vi "Init Chnl from CnfgFile.vi"(8 "error in (no error)":errorcluster, 10 "ChnlSettings":T1={"Channel Name"="", "ChnParameter"={" Delay (µs)"=0.0, "On?"=FALSE, "PositiveVoltage?"=FALSE, "50OhmTerminated? "=FALSE, "25OhmOutput?"=FALSE}, "DelayFormula"="", "OutputModulo"=1, "Go and Done Signal"={"Go Signal"=16, "Done Signal"=16}, "G08_Chnl_Settings"={"Pulse Width (µs)"=0.005, "Output Offset"=0, "Disconnect (E,F)"=FALSE, "Onto MsBus (E,F)"=FALSE, "Input Positive (E,F)"=TRUE, "Param Change"=TRUE, "Inhibit internal clock"=TRUE}} {"ChnParameter"."Delay (µs)" min=0.0 max=100000000.0 format="%.4f"; "G08_Chnl_Settings"."Pulse Width (µs)" min=0.0 max=8947840.0 format="%#.6f"; "Go and Done Signal"."Done Signal" format="%04x" items=["Local Primary"=1, "Local Secondary"=2, "Local Force"=4, "Master Primary"=16]; "Go and Done Signal"."Go Signal" format="%04x" items=["Local Primary0x1"=1, "Local Secondary0x2"=2, "Local Force 0x4"=4, "Resynchronize 0x8"=8, "Master Prim. 0x10"=16, "Master Sec. 0x20"=32, "Master Force  0x40"=64, "System Clock 0x80"=128, "Delay Clock 0x100"=256, "Inhibit Local 0x200"=512, "Start Local 0x400"=1024, "Start Bus 0x800"=2048, "Step Back Local 0x1000"=4096, "Step Back Bus 0x2000"=8192, "RunCircle 0x4000"=16384, "SyncReload 0x8000"=32768, "From E 0x10000"=65536, "From F 0x20000"=131072, "From Bus 0x40000"=262144]}, 11 "BME_DG_G08_Chnl in":refnum<class "BME_DG_G08_Chnl.lvclass">) -> (0 "error out":errorcluster, 3 "BME_DG_G08_Chnl out":refnum<class "BME_DG_G08_Chnl.lvclass">)   [LabVIEW 2009, in "POLARIS BME DG.lvlib" / "BME_DG_G08_Chnl.lvclass"]
uses:
  BME_DG_G08_Chnl.lvclass
  Chnl Settings Complete.ctl
  LV-BME Interface/ChnlSettings.ctl
  Go_Done_Chnl_Settings.ctl
  MSBus.ctl
  SG08_Chnl_Settings.ctl
  BME_DG_G05P2_Chnl/BME_DG_G05P2_Chnl.lvclass
  POLARIS BME DG.lvlib
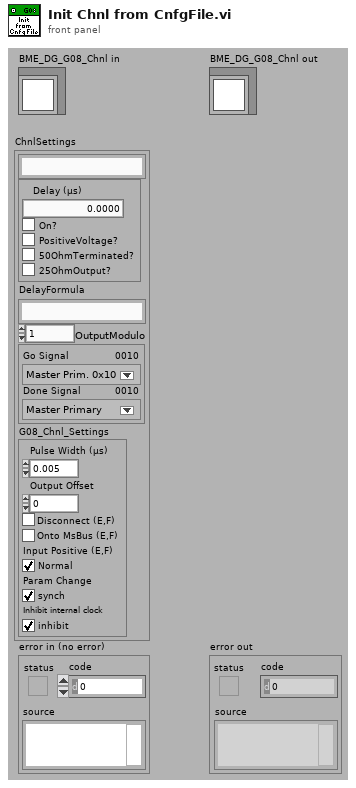
[diagram p1: front panel]
types:
  T1 = typedef "POLARIS BME DG.lvlib/Chnl Settings Complete.ctl" = cluster{"Channel Name":string, "ChnParameter":T2, "DelayFormula":string, "OutputModulo":i32, "Go and Done Signal":T3, "G08_Chnl_Settings":T5}
  T2 = typedef "POLARIS BME DG.lvlib/ChnlSettings.ctl" = cluster{" Delay (µs)":dbl, "On?":bool, "PositiveVoltage?":bool, "50OhmTerminated? ":bool, "25OhmOutput?":bool}
  T3 = typedef "POLARIS BME DG.lvlib/Go_Done_Chnl_Settings.ctl" = cluster{"Go Signal":T4, "Done Signal":u32}
  T4 = typedef "POLARIS BME DG.lvlib/MSBus.ctl" = u32
  T5 = typedef "POLARIS BME DG.lvlib/SG08_Chnl_Settings.ctl" = cluster{"Pulse Width (µs)":dbl, "Output Offset":u32, "Disconnect (E,F)":bool, "Onto MsBus (E,F)":bool, "Input Positive (E,F)":bool, "Param Change":bool, "Inhibit internal clock":bool}
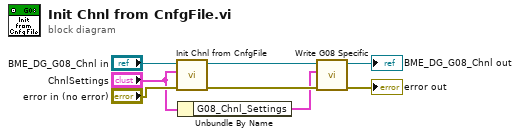
[diagram p0: block diagram]
diagram:
  n1 = call-parent "Init Chnl from CnfgFile.vi"("error in (no error)"="error in (no error)", "ChnlSettings"="ChnlSettings", "BME_DG_G05P2_Chnl in"="BME_DG_G08_Chnl in") -> ("error out"=w5:errorcluster, "BME_DG_G05P2_Chnl out"=w6:refnum<class "BME_DG_G08_Chnl.lvclass">)  [unwired: 7 in]
  n2 = Unbundle By Name("ChnlSettings") -> ("G08_Chnl_Settings"=w1:T5)
  n3 = call-dynamic "Write G08 Specific.vi"("error in (no error)"=w5, "G08_Chnl_Settings"=w1, "BME_DG_G08_Chnl in"=w6) -> ("error out"=→"error out":errorcluster, "BME_DG_G08_Chnl out"=→"BME_DG_G08_Chnl out":refnum<class "BME_DG_G08_Chnl.lvclass">)  [unwired: 7 in]
